vi "Parsing Data.vi"(8 "error in (no error)":errorcluster caption="entrée d'erreur (pas d'erreur)", 11 "Parsing Data RADIO_ERP1 en entrée":refnum<class "Parsing Data RADIO_ERP1.lvclass">) -> (0 "error out":errorcluster caption="sortie d'erreur", 3 "Parsing Data RADIO_ERP1 en sortie":refnum<class "Parsing Data RADIO_ERP1.lvclass">)   [LabVIEW 2020, in "Library Instrument & Equipement.lvlib" / "Library UART.lvlib" / "Parsing Data RADIO_ERP1.lvclass"]
uses:
  Parsing Data RADIO_ERP1.lvclass
  Parsing Data Enocean (Default)/Parsing Data Enocean (Default).lvclass
  Parsing Data RADIO_ERP1.lvclass/Parsing Data RADIO_ERP1.ctl
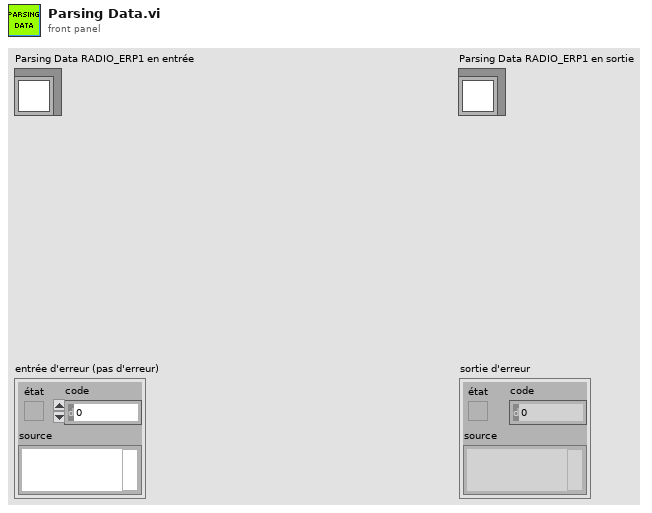
[diagram p1: front panel]
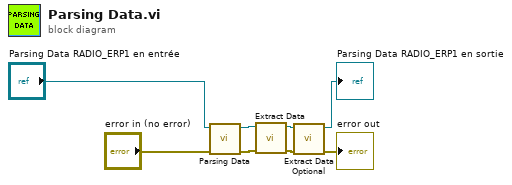
[diagram p0: block diagram]
diagram:
  n1 = call-parent "Parsing Data.vi"("error in (no error)"="error in (no error)", "Parsing Enocean (Default) en entrée"="Parsing Data RADIO_ERP1 en entrée") -> ("error out"=w6:errorcluster, "Parsing Enocean (Default) en sortie"=w5:refnum<class "Parsing Data RADIO_ERP1.lvclass">)  [unwired: 8 in]
  n2 = call-dynamic "Extract Data.vi"("error in (no error)"=w6, "Parsing Data RADIO_ERP1 en entrée"=w5) -> ("error out"=w4:errorcluster, "Parsing Data RADIO_ERP1 en sortie"=w2:refnum<class "Parsing Data RADIO_ERP1.lvclass">)  [unwired: 8 in]
  n3 = call-dynamic "Extract Data Optional.vi"("error in (no error)"=w4, "Parsing Data RADIO_ERP1 en entrée"=w2) -> ("error out"=→"error out":errorcluster, "Parsing Data RADIO_ERP1 en sortie"=→"Parsing Data RADIO_ERP1 en sortie":refnum<class "Parsing Data RADIO_ERP1.lvclass">)  [unwired: 8 in]
